vi "task7.vi"() -> ()   [LabVIEW 2017]
panel:
  out "Value:":string
  in  "Select number system":T1(radio)
  in  "Boolean 7":bool
  in  "Boolean 6":bool
  in  "Boolean 5":bool
  in  "Boolean 4":bool
  in  "Boolean 3":bool
  in  "Boolean 2":bool
  in  "Boolean":bool
  in  "Boolean":bool
  in  "stop":bool
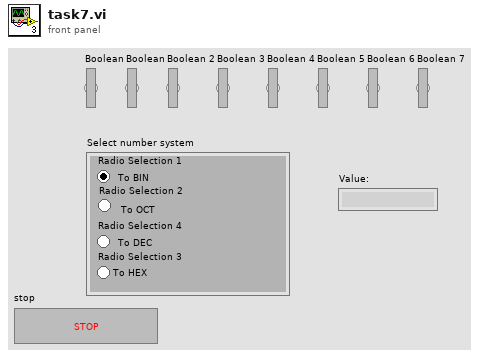
[diagram p1: front panel]
types:
  T1 = enum32{"Radio Selection 1", "Radio Selection 2", "Radio Selection 3", "Radio Selection 4"}
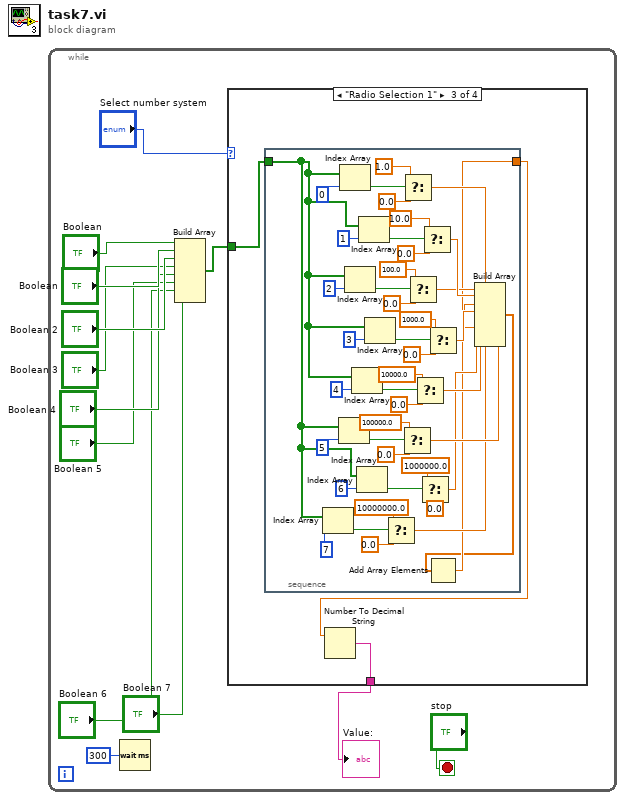
[diagram p0: block diagram]
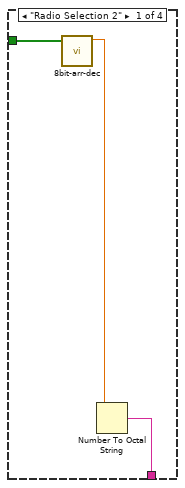
[diagram p2: hidden frame]
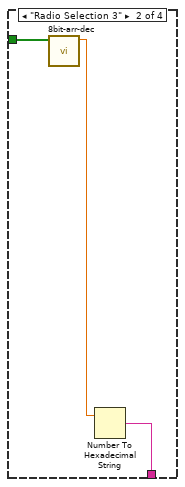
[diagram p3: hidden frame]
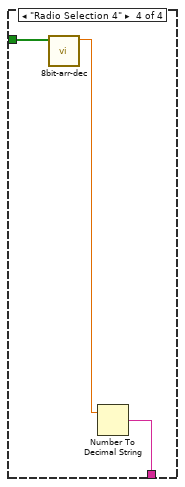
[diagram p4: hidden frame]
diagram:
  n1 = while {
    stop <- "stop" stop-if-true
    n2 = Wait (ms)(milliseconds to wait=u32 300) -> ()  [unwired: 1 out]
    n3 = Build Array("Boolean", "Boolean", "Boolean 2", "Boolean 3", "Boolean 4", "Boolean 5", "Boolean 6", "Boolean 7") -> (w3:bool[])
    n4 = case shown="\"Radio Selection 1\"" "Select number system" {
      tunnel: w3 -> [w16 w19 w22 w68]
      tunnel: [w14 w18 w21 w67] -> w1
      frame "Radio Selection 2" {
        n5 = call "8bit-arr-dec.vi"("Array"=w16) -> ("f"=w15:dbl)  [unwired: 10 in]
        n6 = Number To Octal String(2:w15) -> (0:w14:string)  [unwired: 1 in]
      }
      frame "Radio Selection 3" {
        n7 = call "8bit-arr-dec.vi"("Array"=w19) -> ("f"=w17:dbl)  [unwired: 10 in]
        n8 = Number To Hexadecimal String(2:w17) -> (0:w18:string)  [unwired: 1 in]
      }
      frame "Radio Selection 1" {
        n9 = stacked-sequence {
          tunnel: [w24] -> w20
          tunnel: w22 -> [w33]
          frame #0 {
            n10 = Index Array(array=w33, index=7) -> (element=w34:bool)
            n11 = Index Array(array=w33, index=5) -> (element=w42:bool)
            n12 = Index Array(array=w33, index=0) -> (element=w62:bool)
            n13 = Index Array(array=w33, index=2) -> (element=w54:bool)
            n14 = Index Array(array=w33, index=4) -> (element=w46:bool)
            n15 = Index Array(array=w33, index=6) -> (element=w38:bool)
            n16 = Index Array(array=w33, index=1) -> (element=w58:bool)
            n17 = Index Array(array=w33, index=3) -> (element=w50:bool)
            n18 = Select(t=10000000.0, s=w34, f=0.0) -> (s? t:f=w25:dbl)
            n19 = Select(t=100000.0, s=w42, f=0.0) -> (s? t:f=w27:dbl)
            n20 = Select(t=1.0, s=w62, f=0.0) -> (s? t:f=w32:dbl)
            n21 = Select(t=100.0, s=w54, f=0.0) -> (s? t:f=w30:dbl)
            n22 = Select(t=10000.0, s=w46, f=0.0) -> (s? t:f=w28:dbl)
            n23 = Select(t=1000000.0, s=w38, f=0.0) -> (s? t:f=w26:dbl)
            n24 = Select(t=10.0, s=w58, f=0.0) -> (s? t:f=w31:dbl)
            n25 = Select(t=1000.0, s=w50, f=0.0) -> (s? t:f=w29:dbl)
            n26 = Build Array(w32, w31, w30, w29, w28, w27, w26, w25) -> (w23:dbl[])
            n27 = Add Array Elements(numeric array=w23) -> (sum=w24:dbl)
          }
        }
        n28 = Number To Decimal String(number=w20) -> (decimal integer string=w21:string)  [unwired: 1 in]
      }
      frame "Radio Selection 4" {
        n29 = call "8bit-arr-dec.vi"("Array"=w68) -> ("f"=w66:dbl)  [unwired: 10 in]
        n30 = Number To Decimal String(number=w66) -> (decimal integer string=w67:string)  [unwired: 1 in]
      }
    }
    "Value:" <- w1
  }
